vi "ValveControl_v1.0.vi"() -> ()   [LabVIEW 2015]
panel:
  out "CLOSED":bool
  out "OPEN":bool
  in  "Open Valve":bool
  in  "stop":bool
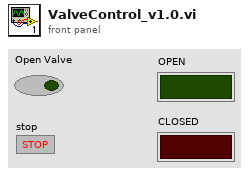
[diagram p1: front panel]
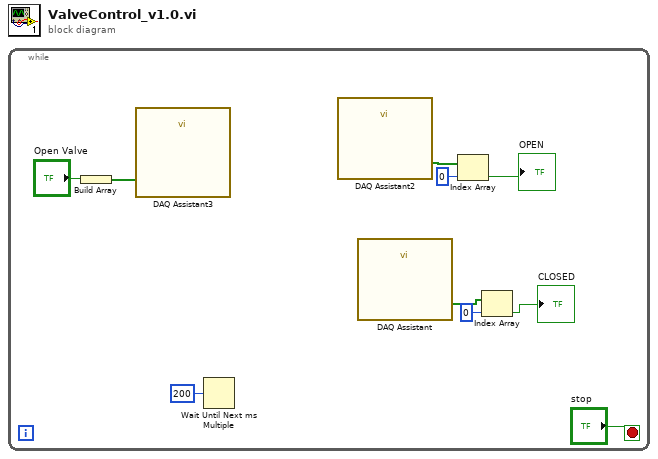
[diagram p0: block diagram]
diagram:
  n1 = while {
    stop <- "stop" stop-if-true
    n2 = Build Array("Open Valve") -> (w7:bool[])
    n3 = call "DAQ Assistant3"("data"=w7) -> ()  [unwired: 17 in, 2 out]
    n4 = Wait Until Next ms Multiple(millisecond multiple=u32 200) -> ()  [unwired: 1 out]
    n5 = call "DAQ Assistant2"() -> ("data"=w4:bool[])  [unwired: 17 in, 2 out]
    n6 = call "DAQ Assistant"() -> ("data"=w6:bool[])  [unwired: 17 in, 2 out]
    n7 = Index Array(array=w4, index=0) -> (element=→"OPEN":bool)
    n8 = Index Array(array=w6, index=0) -> (element=→"CLOSED":bool)
  }
